vi "SystemCore Get Voltage.vi"(11 "error in":errorcluster) -> (4 "input voltage (V)":dbl, 15 "error out":errorcluster)   [LabVIEW 2026, in "MrcLib.lvlib"]
doc: "Returns the input voltage of the SystemCore controller."
uses:
  MrcLib.lvlib
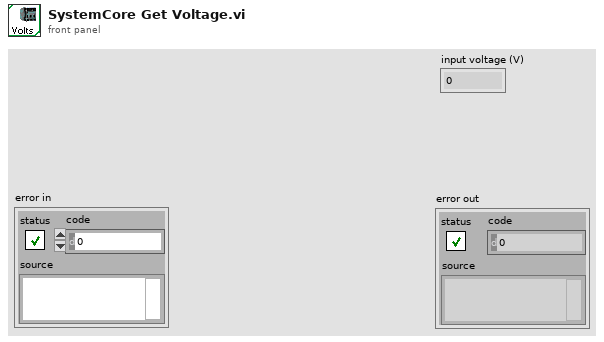
[diagram p1: front panel]
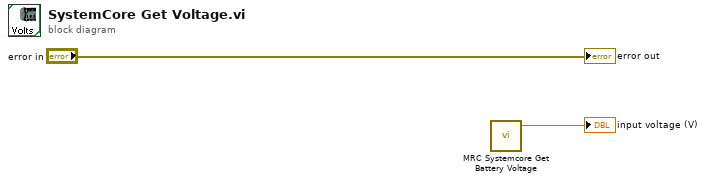
[diagram p0: block diagram]
diagram:
  n1 = call "MRC Systemcore Get Battery Voltage.vi"() -> ("voltage out"=→"input voltage (V)":sgl)  [unwired: 10 in, 1 out]
  "error out" <- "error in"
